vi "AvoidancePolygon.vi"() -> (0 "Polygon":T1)   [LabVIEW 2017]
uses:
  General/PathPlanning/TypeDefs/Polygon2D.ctl
  General/PathPlanning/TypeDefs/Point2D.ctl
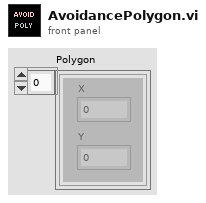
[diagram p1: front panel]
types:
  T1 = typedef "Polygon2D.ctl" = T2[]
  T2 = typedef "Point2D.ctl" = cluster{"X":dbl, "Y":dbl}
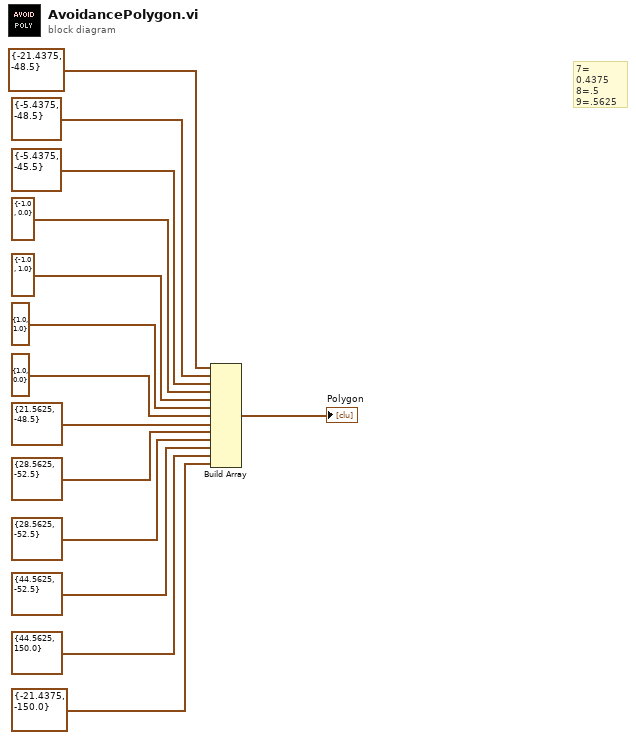
[diagram p0: block diagram]
diagram:
  # "7= 0.4375\n8=.5\n9=.5625"
  n1 = Build Array(T2 {"X"=-21.4375, "Y"=-48.5} ("2DPoint"), T2 {"X"=-5.4375, "Y"=-48.5} ("2DPoint"), T2 {"X"=-5.4375, "Y"=-45.5} ("2DPoint"), T2 {"X"=-1.0, "Y"=0.0} ("2DPoint"), T2 {"X"=-1.0, "Y"=1.0} ("2DPoint"), T2 {"X"=1.0, "Y"=1.0} ("2DPoint"), T2 {"X"=1.0, "Y"=0.0} ("2DPoint"), T2 {"X"=21.5625, "Y"=-48.5} ("2DPoint"), T2 {"X"=28.5625, "Y"=-52.5} ("2DPoint"), T2 {"X"=28.5625, "Y"=-52.5} ("2DPoint"), T2 {"X"=44.5625, "Y"=-52.5} ("2DPoint"), T2 {"X"=44.5625, "Y"=150.0} ("2DPoint"), T2 {"X"=-21.4375, "Y"=-150.0} ("2DPoint")) -> (→"Polygon":T2[])
